vi "Set Detection.vi"(8 "error in (no error)":errorcluster, 10 "Detection":T1=enum."Cy3 (LP550)", 11 "TE2000 in":refnum<class "Eclipse TI.lvclass">) -> (0 "error out":errorcluster, 3 "TE2000 out":refnum<class "Eclipse TI.lvclass">)   [LabVIEW 2015, in "Eclipse TI.lvlib" / "Eclipse TI.lvclass"]
uses:
  Eclipse TI.lvclass
  Resources/Type Defs/Detection.ctl
  Eclipse TI.lvclass/Eclipse TI.ctl
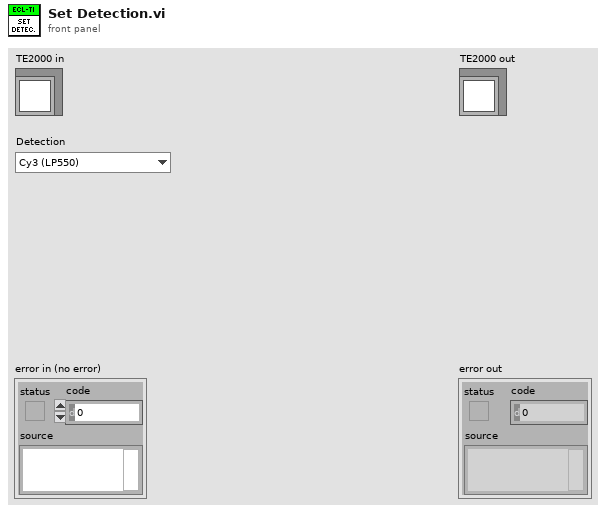
[diagram p1: front panel]
types:
  T1 = typedef "Detection.ctl" = enum16{"Cy2 (LP500)", "Cy3 (LP550)", "Cy5 (BP700/75)", "Cy3/Cy5 (BP590/40,700/60)", "No Filter", "Laser to Eyes"}
  T2 = typedef "Microscope Type.ctl" = enum16{"TE2000", "Eclipse Ti"}
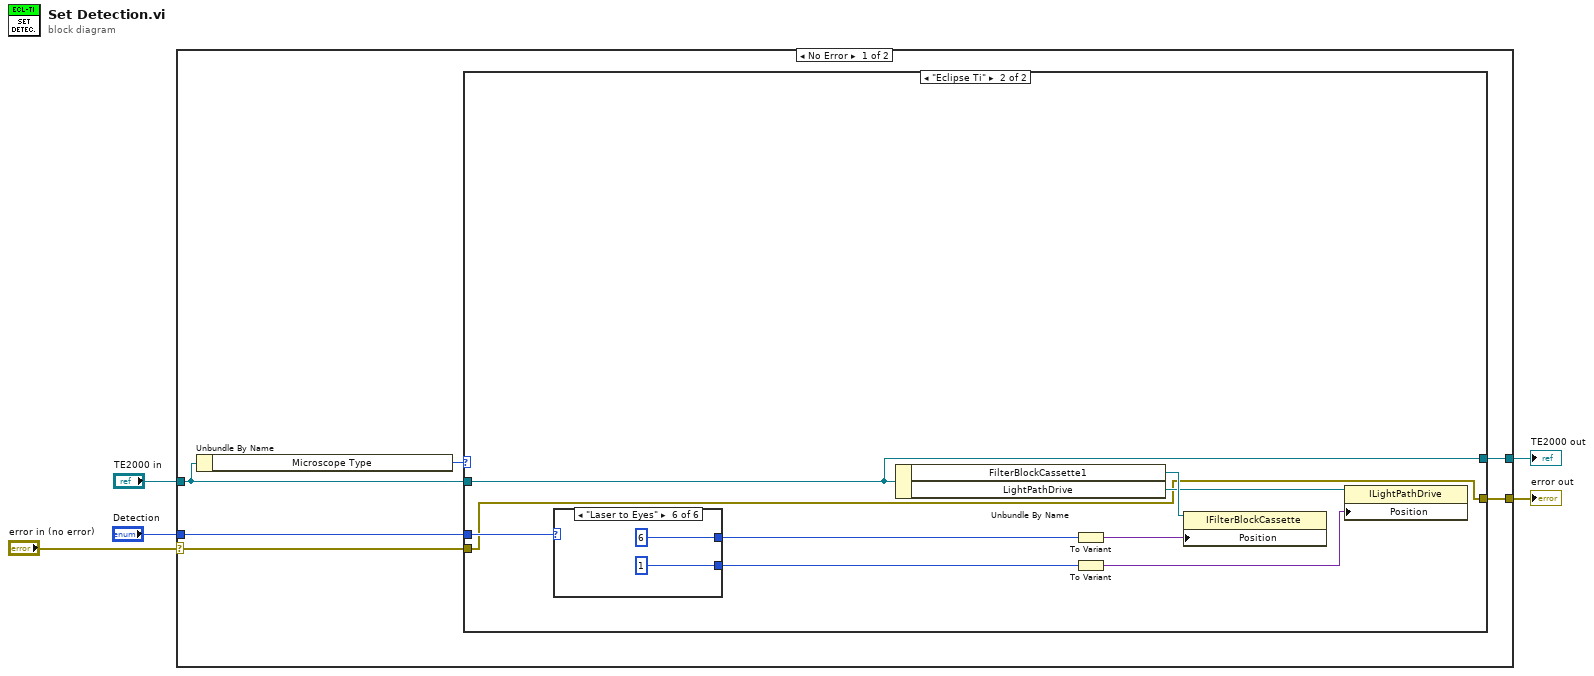
[diagram p0: block diagram]
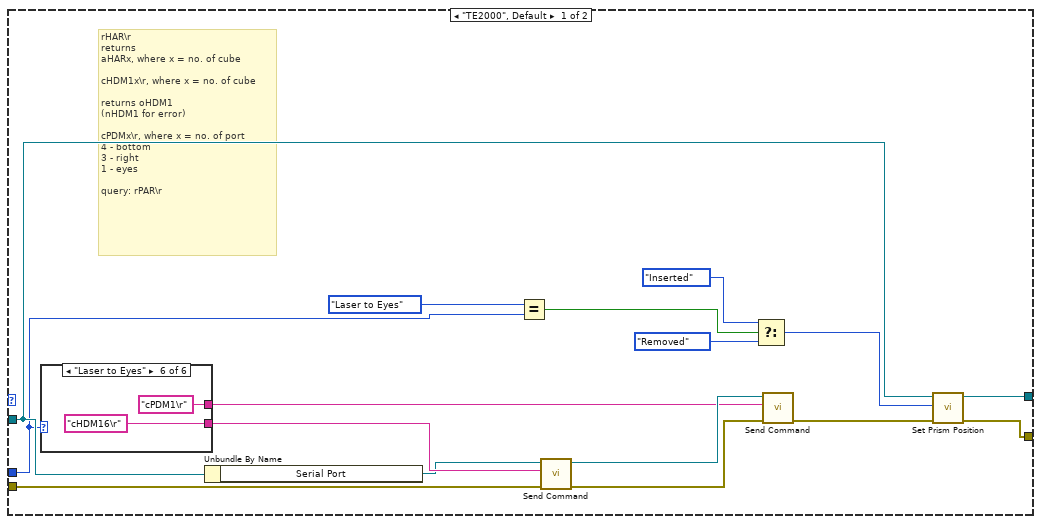
[diagram p2: hidden frame]
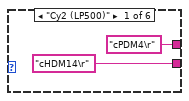
[diagram p3: hidden frame]
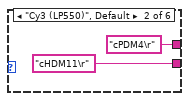
[diagram p4: hidden frame]
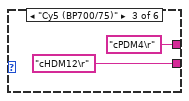
[diagram p5: hidden frame]
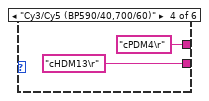
[diagram p6: hidden frame]
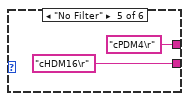
[diagram p7: hidden frame]
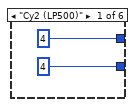
[diagram p8: hidden frame]
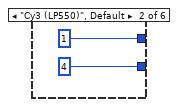
[diagram p9: hidden frame]
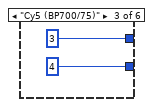
[diagram p10: hidden frame]
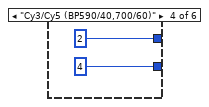
[diagram p11: hidden frame]
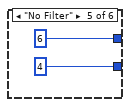
[diagram p12: hidden frame]
diagram:
  n1 = case shown="No Error" "error in (no error)" {
    selector: "error in (no error)" -> [w11 w62]
    tunnel: [w10 w62] -> w4
    tunnel: [w9 w61] -> w2
    tunnel: "TE2000 in" -> [w7 w61]
    tunnel: "Detection" -> [w8 _]
    frame No Error {
      n2 = Unbundle By Name(w7) -> ("Microscope Type"=w6:T2)
      n3 = case shown="\"Eclipse Ti\"" w6 {
        tunnel: w11 -> [w27 w40]
        tunnel: [w20 w40] -> w10
        tunnel: w7 -> [w19 w41]
        tunnel: [w18 w41] -> w9
        tunnel: w8 -> [w17 w48]
        frame "TE2000", Default {
          # "rHAR\\r\nreturns\naHARx, where x = no. of cube\n\ncHDM1x\\r, where x = no. of cube\n\nreturns oHDM1\n(nHDM1 for error)\n\ncPDMx\\r, where x = no. of port\n4 - bottom\n3 - right\n1 - eyes\n\nquery: rPAR\\r"
          n4 = case shown="\"Laser to Eyes\"" w17 {
            tunnel: ["cHDM14\r" "cHDM11\r" "cHDM12\r" "cHDM13\r" "cHDM16\r" "cHDM16\r"] -> w24
            tunnel: ["cPDM4\r" "cPDM4\r" "cPDM4\r" "cPDM4\r" "cPDM4\r" "cPDM1\r"] -> w23
            frame "Cy2 (LP500)" {
            }
            frame "Cy3 (LP550)", Default {
            }
            frame "Cy5 (BP700/75)" {
            }
            frame "Cy3/Cy5 (BP590/40,700/60)" {
            }
            frame "No Filter" {
            }
            frame "Laser to Eyes" {
            }
          }
          n5 = Unbundle By Name(w19) -> ("Serial Port"=w22:refnum<visa-resource-name>)
          n6 = Equal?(x=Detection."Laser to Eyes", y=w17) -> (x = y?=w15:bool)
          n7 = call "Send Command.vi"("error in (no error)"=w27, "Command"=w24, "Serial Port In"=w22) -> ("error out"=w26:errorcluster, "Serial Port Out"=w25:refnum<visa-resource-name>)  [unwired: 6 in, 1 out]
          n8 = Select(t=enum16{"Removed", "Inserted"}."Inserted" ("Prism Position"), s=w15, f=enum16{"Removed", "Inserted"}."Removed" ("Prism Position")) -> (s? t:f=w12:enum16{"Removed", "Inserted"})
          n9 = call "Send Command.vi"("error in (no error)"=w26, "Command"=w23, "Serial Port In"=w25) -> ("error out"=w21:errorcluster)  [unwired: 6 in, 2 out]
          n10 = call-dynamic "Set Prism Position.vi"("error in (no error)"=w21, "Prism Position"=w12, "TE2000 in"=w19) -> ("error out"=w20:errorcluster, "TE2000 out"=w18:refnum<class "Eclipse TI.lvclass">)  [unwired: 7 in]
        }
        frame "Eclipse Ti" {
          n11 = case shown="\"Laser to Eyes\"" w48 {
            tunnel: [4 4 4 4 4 1] -> w43
            tunnel: [4 1 3 2 6 6] -> w42
            frame "Cy2 (LP500)" {
            }
            frame "Cy3 (LP550)", Default {
            }
            frame "Cy5 (BP700/75)" {
            }
            frame "Cy3/Cy5 (BP590/40,700/60)" {
            }
            frame "No Filter" {
            }
            frame "Laser to Eyes" {
            }
          }
          n12 = Unbundle By Name(w41) -> ("FilterBlockCassette1"=w45:refnum<k7>, "LightPathDrive"=w44:refnum<k7>)
          n13 = To Variant(anything=w42) -> (Variant=w46:variant)
          n14 = To Variant(anything=w43) -> (Variant=w47:variant)
          n15 = property class="IFilterBlockCassette"(reference=w45, "Position"=w46) -> ()  [unwired: 1 in, 2 out]
          n16 = property class="ILightPathDrive"(reference=w44, "Position"=w47) -> ()  [unwired: 1 in, 2 out]
        }
      }
    }
    frame Error {
    }
  }
  "error out" <- w4
  "TE2000 out" <- w2
